vi "TestVirtual1.vi"(0 "reference in":refnum<class "G#SubClass2.lvclass">, 5 "error in (no error)":errorcluster) -> (14 "reference out":refnum<class "G#SubClass2.lvclass">, 15 "MethodName":string[](array[string]), 19 "error out":errorcluster)   [LabVIEW 2017, in "G#SubClass2.lvclass"]
uses:
  G#SubClass2.lvclass
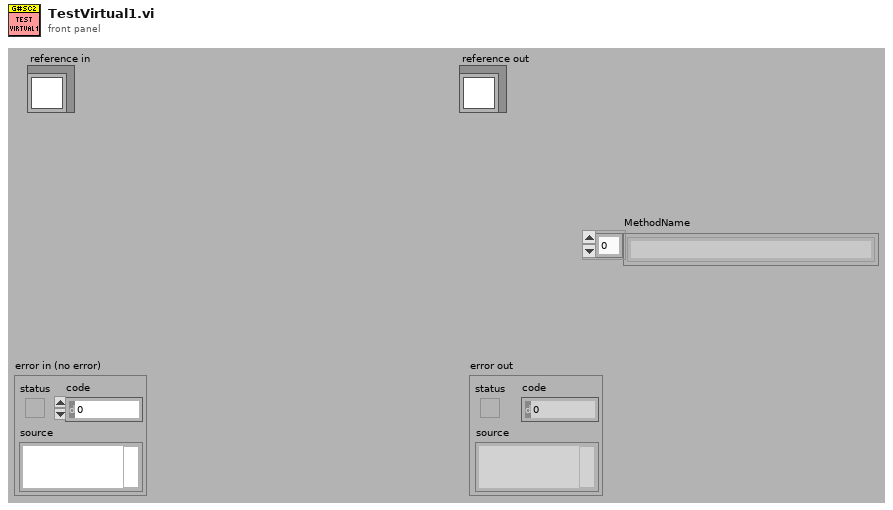
[diagram p1: front panel]
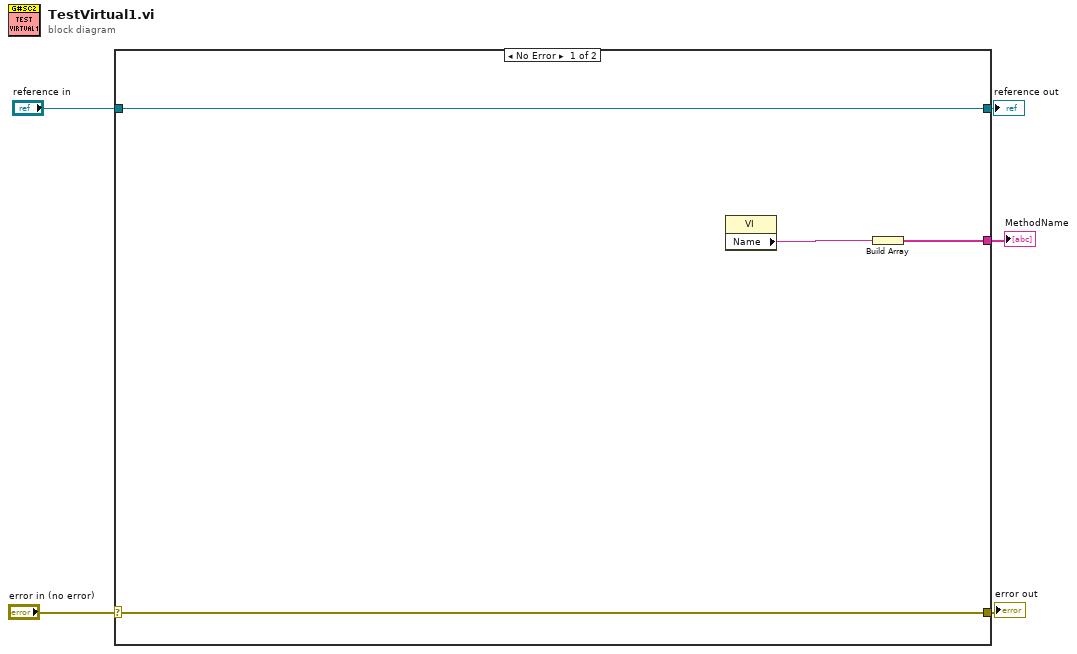
[diagram p0: block diagram]
diagram:
  n1 = case shown="No Error" "error in (no error)" {
    selector: "error in (no error)" -> [w9 w11]
    tunnel: [w9 w11] -> w4
    tunnel: [w8 w10] -> w2
    tunnel: "reference in" -> [w8 w10]
    tunnel: [w6 _] -> w1
    frame No Error {
      n2 = property class="VI"() -> ("Name"=w7:string)  [unwired: 2 in, 2 out]
      n3 = Build Array(w7) -> (w6:string[])
    }
    frame Error {
    }
  }
  "error out" <- w4
  "reference out" <- w2
  "MethodName" <- w1
